vi "Collect_Beam_Positions.vi"(1 "Align Probe Using":enum16{"Green Beams", "Blue Beams"}(ring), 2 "Use Specification Beam Half-Angle":bool) -> ()   [LabVIEW 2012]
uses:
  Controls/Tunnel_Coordinates.ctl
  Gen Trav/Trav_mode.ctl
  Controls/User_Specific_mode.ctl
  Globals/Trav_pos_global.vi
  Globals/Preference_global.vi
  Globals/Constants_global.vi
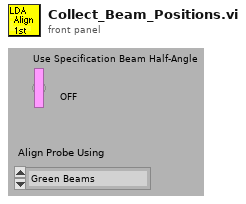
[diagram p1: front panel]
types:
  T1 = typedef "Tunnel_Coordinates.ctl" = enum16{"Work in Tunnel Coordinates", "Work in Model Coordinates"}
  T2 = typedef "User_Specific_mode.ctl" = enum16{"Check VI only", "Run VI"}
  T3 = typedef "Trav_mode.ctl" = enum16{"Move traverse", "Read traverse position", "Teach Position"}
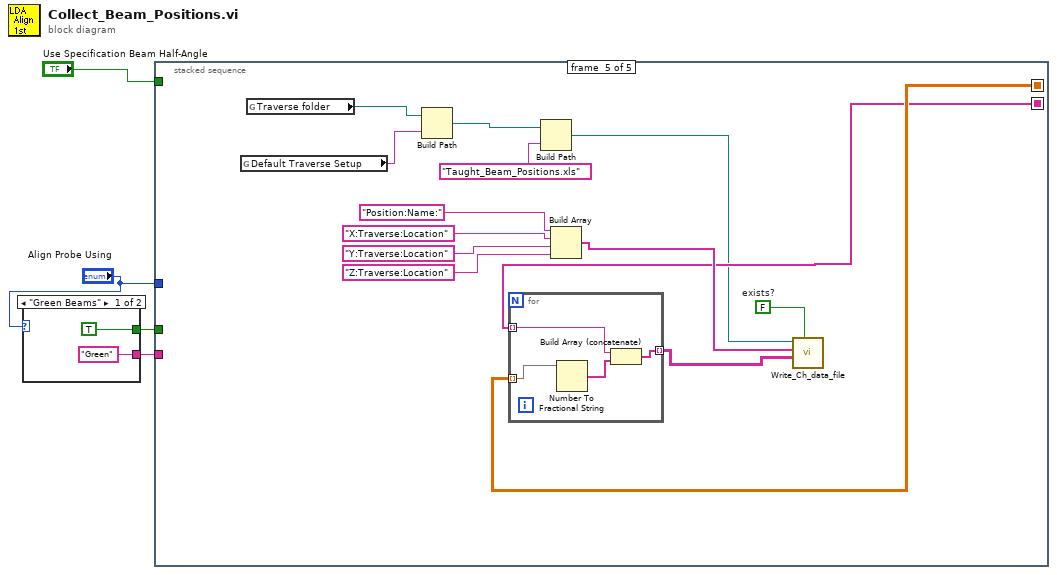
[diagram p0: block diagram]
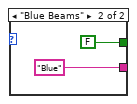
[diagram p2: hidden frame]
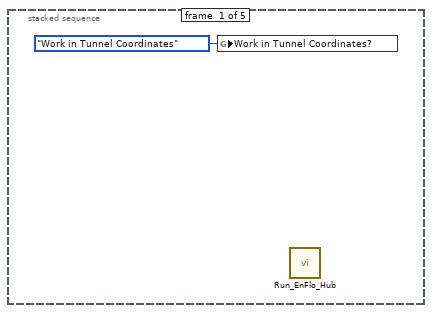
[diagram p3: hidden frame]
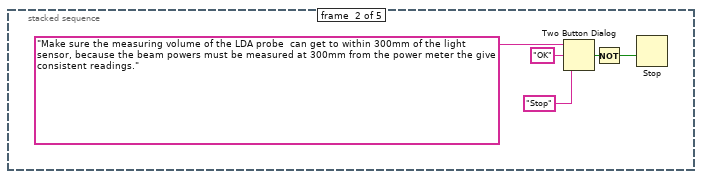
[diagram p4: hidden frame]
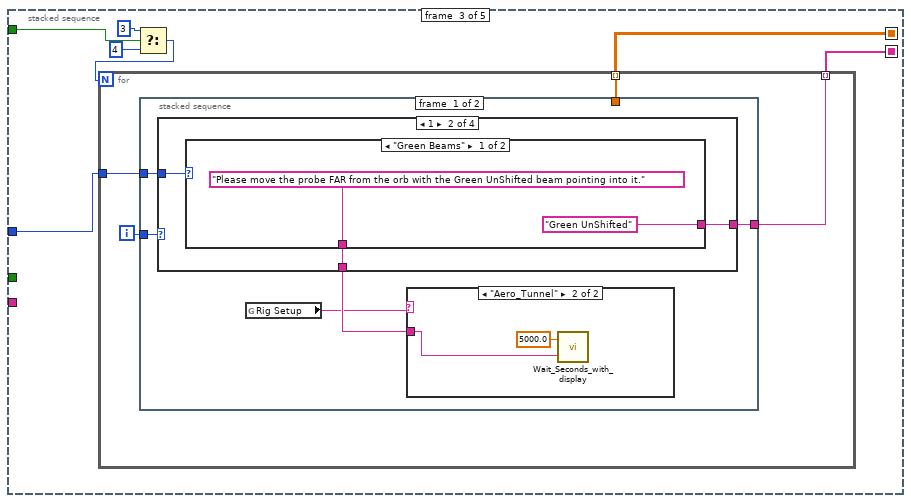
[diagram p5: hidden frame]
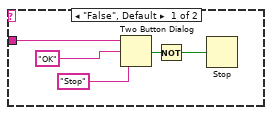
[diagram p6: hidden frame]
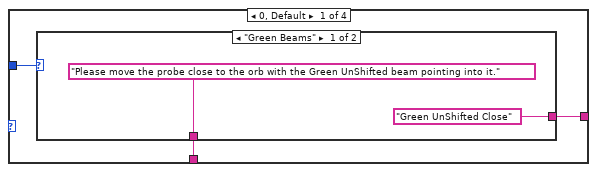
[diagram p7: hidden frame]
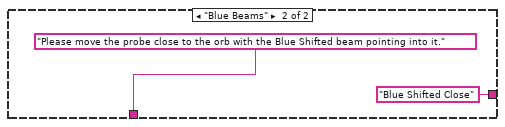
[diagram p8: hidden frame]
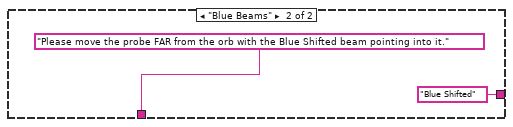
[diagram p9: hidden frame]
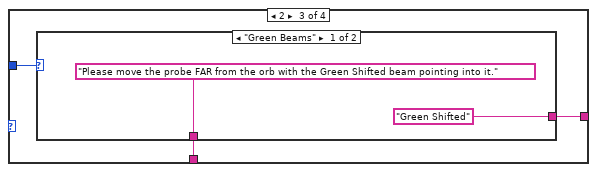
[diagram p10: hidden frame]
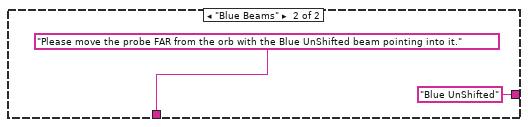
[diagram p11: hidden frame]
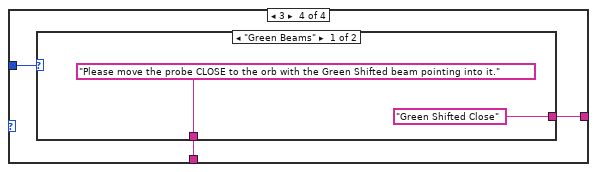
[diagram p12: hidden frame]
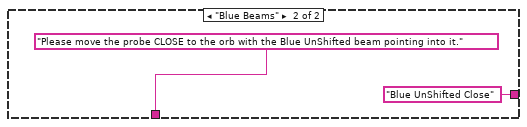
[diagram p13: hidden frame]
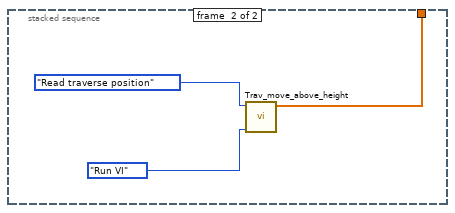
[diagram p14: hidden frame]
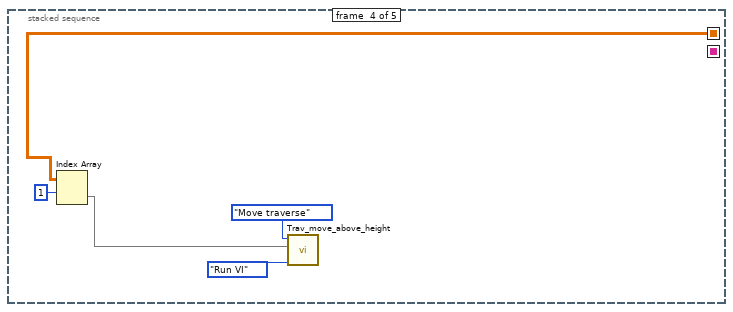
[diagram p15: hidden frame]
diagram:
  n1 = case shown="\"Green Beams\"" "Align Probe Using" {
    tunnel: [TRUE FALSE] -> w4
    tunnel: ["Green" "Blue"] -> w1
    frame "Green Beams" {
    }
    frame "Blue Beams" {
    }
  }
  n2 = stacked-sequence {
    seq-local: [_ _ w16 _ _] -> [_ _ _ w71 w77]
    seq-local: [_ _ w15 _ _] -> [_ _ _ _ w76]
    tunnel: w4 -> [_ _ _ _ _]
    tunnel: "Use Specification Beam Half-Angle" -> [_ _ w20 _ _]
    tunnel: "Align Probe Using" -> [_ _ w21 _ _]
    tunnel: w1 -> [_ _ _ _ _]
    frame #0 {
      n3 = global write "Trav_pos_global.vi" "Work in Tunnel Coordinates?"(Tunnel_Coordinates."Work in Tunnel Coordinates" ("Work in Tunnel Coordinates?")) -> ()
      n4 = call "Run_EnFlo_Hub.vi"() -> ()  [unwired: 8 out]
    }
    frame #1 {
      n5 = Two Button Dialog(message="Make sure the measuring volume of the LDA probe  can get to within 300mm of the light sensor, because the beam powers must be measured at 300mm from the power meter the give consistent readings.", 1:"Stop" ("F button name (\"Cancel\")"), 2:"OK" ("T button name (\"OK\")")) -> (T button?=w11:bool)
      n6 = Not(x=w11) -> (.not. x?=w10:bool)
      n7 = Stop(stop? (T)=w10) -> ()
    }
    frame #2 {
      n8 = Select(t=3, s=w20, f=4) -> (s? t:f=w17:i32)
      n9 = for {
        N: w17 -> [_]
        tunnel: [w25] -> w16 mode=indexing
        tunnel: w21 -> [w24]
        tunnel: [w23] -> w15 mode=indexing
        i -> [w22]
        n10 = stacked-sequence {
          tunnel: [_ w66] -> w25
          tunnel: w24 -> [w29 _]
          tunnel: [w28 _] -> w23
          tunnel: w22 -> [w27 _]
          frame #0 {
            n11 = case shown="1" w27 {
              tunnel: [w40 w47 w54 w61] -> w30
              tunnel: w29 -> [w39 w46 w53 w60]
              tunnel: [w38 w45 w52 w59] -> w28
              frame 0, Default {
                n12 = case shown="\"Green Beams\"" w39 {
                  tunnel: ["Please move the probe close to the orb with the Green UnShifted beam pointing into it." ("message") "Please move the probe close to the orb with the Blue Shifted beam pointing into it." ("message")] -> w40
                  tunnel: ["Green UnShifted Close" "Blue Shifted Close"] -> w38
                  frame "Green Beams" {
                  }
                  frame "Blue Beams" {
                  }
                }
              }
              frame 1 {
                n13 = case shown="\"Green Beams\"" w46 {
                  tunnel: ["Please move the probe FAR from the orb with the Green UnShifted beam pointing into it." ("message") "Please move the probe FAR from the orb with the Blue Shifted beam pointing into it." ("message")] -> w47
                  tunnel: ["Green UnShifted" "Blue Shifted"] -> w45
                  frame "Green Beams" {
                  }
                  frame "Blue Beams" {
                  }
                }
              }
              frame 2 {
                n14 = case shown="\"Green Beams\"" w53 {
                  tunnel: ["Please move the probe FAR from the orb with the Green Shifted beam pointing into it." ("message") "Please move the probe FAR from the orb with the Blue UnShifted beam pointing into it." ("message")] -> w54
                  tunnel: ["Green Shifted" "Blue UnShifted"] -> w52
                  frame "Green Beams" {
                  }
                  frame "Blue Beams" {
                  }
                }
              }
              frame 3 {
                n15 = case shown="\"Green Beams\"" w60 {
                  tunnel: ["Please move the probe CLOSE to the orb with the Green Shifted beam pointing into it." ("message") "Please move the probe CLOSE to the orb with the Blue UnShifted beam pointing into it." ("message")] -> w61
                  tunnel: ["Green Shifted Close" "Blue UnShifted Close"] -> w59
                  frame "Green Beams" {
                  }
                  frame "Blue Beams" {
                  }
                }
              }
            }
            n16 = global read "Preference_global.vi" "Rig Setup"() -> (w26:string)
            n17 = case shown="\"Aero_Tunnel\"" w26 {
              tunnel: w30 -> [w35 w36]
              frame "False", Default {
                n18 = Two Button Dialog(message=w35, 1:"Stop" ("F button name (\"Cancel\")"), 2:"OK" ("T button name (\"OK\")")) -> (T button?=w32:bool)
                n19 = Not(x=w32) -> (.not. x?=w31:bool)
                n20 = Stop(stop? (T)=w31) -> ()
              }
              frame "Aero_Tunnel" {
                n21 = call "Wait_Seconds_with_display.vi"("Message"=w36, "Seconds to wait"=5000.0) -> ()  [unwired: 1 in, 1 out]
              }
            }
          }
          frame #1 {
            n22 = call "Trav_move_above_height.vi"("Simulate/Run"=User_Specific_mode."Run VI", "Mode"=Trav_mode."Read traverse position") -> ("Trav Position achieved"=w66:dbl[])  [unwired: 5 in, 4 out]
          }
        }
      }
    }
    frame #3 {
      n23 = Index Array(array=w71, index (row)=1) -> (element=w69:dbl[])  [unwired: 1 in]
      n24 = call "Trav_move_above_height.vi"("Simulate/Run"=User_Specific_mode."Run VI", "New Position"=w69, "Mode"=Trav_mode."Move traverse") -> ()  [unwired: 4 in, 5 out]
    }
    frame #4 {
      w79 = FALSE  # exists?
      n25 = global read "Trav_pos_global.vi" "Default Traverse Setup"() -> (w86:string)
      n26 = global read "Constants_global.vi" "Traverse folder"() -> (w84:path)
      n27 = Build Path(base path=w84, name or relative path=w86) -> (appended path=w85:path)
      n28 = for {
        tunnel: w77 -> [w91] mode=indexing
        tunnel: w76 -> [w90] mode=indexing
        tunnel: [w88] -> w75 mode=indexing
        n29 = Number To Fractional String(number=w91) -> (F-format string=w89:string[])  [unwired: 3 out]
        n30 = Build Array (concatenate)(w90, w89) -> (w88:string[])
      }
      n31 = Build Path(base path=w85, name or relative path="Taught_Beam_Positions.xls" ("Substring")) -> (appended path=w74:path)
      n32 = Build Array("Position:Name:", "X:Traverse:Location", "Y:Traverse:Location", "Z:Traverse:Location") -> (w78:string[])
      n33 = call "Write_Ch_data_file.vi"("exists?"=w79, "Channel Values"=w75, "Channel names"=w78, "Filename"=w74) -> ()  [unwired: 4 in, 4 out]
    }
  }
